vi "Lancing_Presence_Absence.vi"(0 "Ref ROI Parameters":T5={"Ref ROI"={"Global Rectangle"=[], "Contours"=[]}, "Ref ROI Edge Options"={"Edge Polarity"=2, "Kernel Size"=3, "Width"=3, "Minimum Edge Strength"=50.0, "Interpolation Type"=enum."Zero Order", "Data Processing Method"=enum."Average"}, "Ref ROI Line Options"={"Number of Lines"=1, "Type"=enum."Best Edge Rake", "Min. Score"=10.0, "Max. Score"=1000.0, "Orientation"=0.0, "Angle Range"=10.0, "Angle Tolerance"=10.0, "Step Size"=8, "Min. SNR (db)"=0.0, "Min. Points (%)"=25.0, "Hough Iterations"=5}, "Ref ROI Search Direction"=0, "Ref ROI Overlay"=FALSE, "Ref Edge/Point Overlay"=FALSE, "Ref ROI Rake Line Overlay"=FALSE} {"Ref ROI Search Direction" items=["Left to Right", "Right to Left", "Top to Bottom", "Bottom to Top"]; "Ref ROI Line Options"."Min. Points (%)" min=0.0 max=100.0; "Ref ROI Line Options"."Min. SNR (db)" min=0.0; "Ref ROI Line Options"."Max. Score" min=0.0 max=1024.0; "Ref ROI Line Options"."Min. Score" min=0.0 max=1024.0 step=1.0; "Ref ROI Edge Options"."Edge Polarity" items=["All Edges", "Rising Edges", "Falling Edges"]; "Ref ROI Edge Options"."Minimum Edge Strength" format="%.2f"; "Ref ROI Edge Options"."Width" step=2; "Ref ROI Edge Options"."Kernel Size" step=2; "Ref ROI"."Contours"."Type" items=["No Selection", "Point", "Line", "Rectangle", "Oval", "Polygon", "Free", "Annulus", "Unused2", "Unused3", "Broken Line", "Free Hand Line", "Rotated Rectangle"]}, 1 "Calibrated Image":T8, 5 "ROI 1 Parameters":T7={"ROI 1[Before Transformation]"={"Global Rectangle"=[], "Contours"=[]}, "ROI 1 Edge Options"={"Edge Polarity"=2, "Kernel Size"=3, "Width"=3, "Minimum Edge Strength"=50.0, "Interpolation Type"=enum."Zero Order", "Data Processing Method"=enum."Average"}, "ROI 1 Process"=enum."Get First + Last Edge", "ROI 1 Step Size"=4, "ROI 1 Scan Direction"=3, "ROI 1 Overlay"=FALSE, "ROI 1 Rake Line Overlay"=FALSE, "ROI 1 Edge/Point Overlay "=FALSE} {"ROI 1 Scan Direction" items=["Left To Right", "Right To Left", "Top To Bottom", "Bottom To Top"]; "ROI 1 Edge Options"."Edge Polarity" items=["All Edges", "Rising Edges", "Falling Edges"]; "ROI 1 Edge Options"."Minimum Edge Strength" format="%.2f"; "ROI 1 Edge Options"."Width" step=2; "ROI 1 Edge Options"."Kernel Size" step=2}, 7 "ROI 2 Parameters":T6={"ROI 2 Edge Options"={"Edge Polarity"=2, "Kernel Size"=3, "Width"=3, "Minimum Edge Strength"=50.0, "Interpolation Type"=enum."Zero Order", "Data Processing Method"=enum."Average"}, "ROI 2 Scan Direction"=3, "ROI 2 Step Size"=3, "ROI 2 Process"=enum."Get First + Last Edge", "ROI 2 Overlay"=FALSE, "ROI 2 Rake Line Overlay"=FALSE, "ROI 2 Edge/Point Overlay "=FALSE} {"ROI 2 Scan Direction" items=["Left To Right", "Right To Left", "Top To Bottom", "Bottom To Top"]; "ROI 2 Edge Options"."Edge Polarity" items=["All Edges", "Rising Edges", "Falling Edges"]; "ROI 2 Edge Options"."Minimum Edge Strength" format="%.2f"; "ROI 2 Edge Options"."Width" step=2; "ROI 2 Edge Options"."Kernel Size" step=2}, 9 "Image In":T8(plugin-control), 11 "error in (no error)":errorcluster, 12 "Ellipse Center":cluster{"Center X":dbl, "Center Y":dbl}) -> (4 "Points for Arrow Overlay":cluster{"X":sgl, "Y":sgl}[](array[cluster]), 6 "Value":dbl, 8 "Height 2":sgl, 15 "error out":errorcluster)   [LabVIEW 2019, in "Algorithm.lvclass"]
uses:
  FrameworkOverrides/Algorithm.lvclass
  <vilib>/vision/NI_Vision_Development_Module.lvlib
  <vilib>/vision/Measure.llb/Edge Polarity.ctl
  <vilib>/vision/Measure.llb/Edge Options.ctl
  <vilib>/vision/Image Controls.llb/IMAQ Image.ctl
  <vilib>/vision/Measure.llb/Straight Edge Process.ctl
  <vilib>/vision/Measure.llb/Straight Edge Options.ctl
panel:
  out "Height":sgl
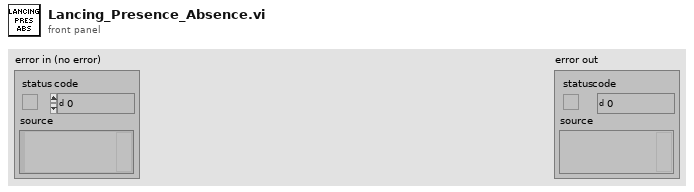
[diagram p1: front panel]
types:
  T1 = typedef "Edge Options.ctl" = cluster{"Edge Polarity":T2, "Kernel Size":u32, "Width":u32, "Minimum Edge Strength":sgl, "Interpolation Type":enum32{"Zero Order", "Bilinear", "Quadratic", "Cubic", "Bilinear Fixed"}, "Data Processing Method":enum32{"Average", "Median"}}
  T2 = typedef "Edge Polarity.ctl" = u32
  T3 = typedef "Straight Edge Options.ctl" = cluster{"Number of Lines":i32, "Type":T4, "Min. Score":dbl, "Max. Score":dbl, "Orientation":dbl, "Angle Range":dbl, "Angle Tolerance":dbl, "Step Size":u32, "Min. SNR (db)":dbl, "Min. Points (%)":dbl, "Hough Iterations":i32}
  T4 = typedef "Straight Edge Process.ctl" = enum32{"First Edge Rake", "Best Edge Rake", "Hough Edge Rake", "First Edge Projection", "Best Edge Projection"}
  T5 = cluster{"Ref ROI":cluster{"Global Rectangle":i32[], "Contours":cluster{"ID":enum32{"External", "Internal"}, "Type":u32, "Coordinates":i32[]}[]}, "Ref ROI Edge Options":T1, "Ref ROI Line Options":T3, "Ref ROI Search Direction":u32, "Ref ROI Overlay":bool, "Ref Edge/Point Overlay":bool, "Ref ROI Rake Line Overlay":bool}
  T6 = cluster{"ROI 2 Edge Options":T1, "ROI 2 Scan Direction":u16, "ROI 2 Step Size":u32, "ROI 2 Process":enum16{"Get First Edge", "Get First + Last Edge", "Get All Edges", "Get Best Edge"}, "ROI 2 Overlay":bool, "ROI 2 Rake Line Overlay":bool, "ROI 2 Edge/Point Overlay ":bool}
  T7 = cluster{"ROI 1[Before Transformation]":cluster{"Global Rectangle":i32[], "Contours":cluster{"Contour Type":u32, "ROI Type":u32, "Points":i32[]}[]}, "ROI 1 Edge Options":T1, "ROI 1 Process":enum16{"Get First Edge", "Get First + Last Edge", "Get All Edges", "Get Best Edge"}, "ROI 1 Step Size":u32, "ROI 1 Scan Direction":u16, "ROI 1 Overlay":bool, "ROI 1 Rake Line Overlay":bool, "ROI 1 Edge/Point Overlay ":bool}
  T8 = typedef "IMAQ Image.ctl" = refnum<image>
  T9 = cluster{"Left":dbl, "Top":dbl, "Right":dbl, "Bottom":dbl, "Angle":dbl}
  T10 = typedef "IMAQ Rectangle" = cluster{"Left":i32, "Top":i32, "Right":i32, "Bottom":i32, "Rotation":dbl}
  T11 = cluster{"Global Rectangle":i32[], "Contours":cluster{"ID":enum32{"External", "Internal"}, "Type":u32, "Coordinates":i32[]}[]}
  T12 = cluster{"ID":enum32{"External", "Internal"}, "Type":u32, "Coordinates":i32[]}[]
  T13 = cluster{"ID":enum32{"External", "Internal"}, "Type":u32, "Coordinates":i32[]}
  T14 = cluster{"Coordinates[0]":i32, "Coordinates[1]":i32, "Coordinates[2]":i32, "Coordinates[3]":i32, "Coordinates[4]":i32}
  T15 = typedef "ROI Descriptor" = cluster{"Global Rectangle":i32[], "Contours":cluster{"ID":enum32{"External", "Internal"}, "Type":u32, "Coordinates":i32[]}[]}
  T16 = cluster{"Global Rectangle":i32[], "Contours":cluster{"Contour Type":u32, "ROI Type":u32, "Points":i32[]}[]}
  T17 = enum16{"Get First Edge", "Get First + Last Edge", "Get All Edges", "Get Best Edge"}
  T18 = cluster{"Contour Type":u32, "ROI Type":u32, "Points":i32[]}[]
  T19 = cluster{"Contour Type":u32, "ROI Type":u32, "Points":i32[]}
  T20 = cluster{"Points[0]":i32, "Points[1]":i32, "Points[2]":i32, "Points[3]":i32, "Points[4]":i32}
  T21 = cluster{"Point1 (Pixels)":cluster{"X":sgl, "Y":sgl}, "Point2 (Pixels)":cluster{"X":sgl, "Y":sgl}, "Point1 (Real-World)":cluster{"X":sgl, "Y":sgl}, "Point2 (Real-World)":cluster{"X":sgl, "Y":sgl}, "Angle (Pixel)":dbl, "Angle (Real-World)":dbl, "Score":dbl, "Straightness":dbl, "Average SNR (db)":dbl, "Calibration Valid":bool}[]
  T22 = typedef "Search Line.ctl" = cluster{"Start Point":cluster{"X":sgl, "Y":sgl}, "End Point":cluster{"X":sgl, "Y":sgl}, "Edge Info":T23[], "Edge Map":dbl[], "Calibration Valid":bool}
  T23 = typedef "Edge New.ctl" = cluster{"Location (Pixel)":cluster{"X":sgl, "Y":sgl}, "Location (Real-World)":cluster{"X":sgl, "Y":sgl}, "Distance (Pixel)":dbl, "Distance (Real-World)":dbl, "Strength":dbl, "Noise":dbl, "Rising?":bool}
  T24 = cluster{"Point1 (Pixels)":cluster{"X":sgl, "Y":sgl}, "Point2 (Pixels)":cluster{"X":sgl, "Y":sgl}, "Point1 (Real-World)":cluster{"X":sgl, "Y":sgl}, "Point2 (Real-World)":cluster{"X":sgl, "Y":sgl}, "Angle (Pixel)":dbl, "Angle (Real-World)":dbl, "Score":dbl, "Straightness":dbl, "Average SNR (db)":dbl, "Calibration Valid":bool}
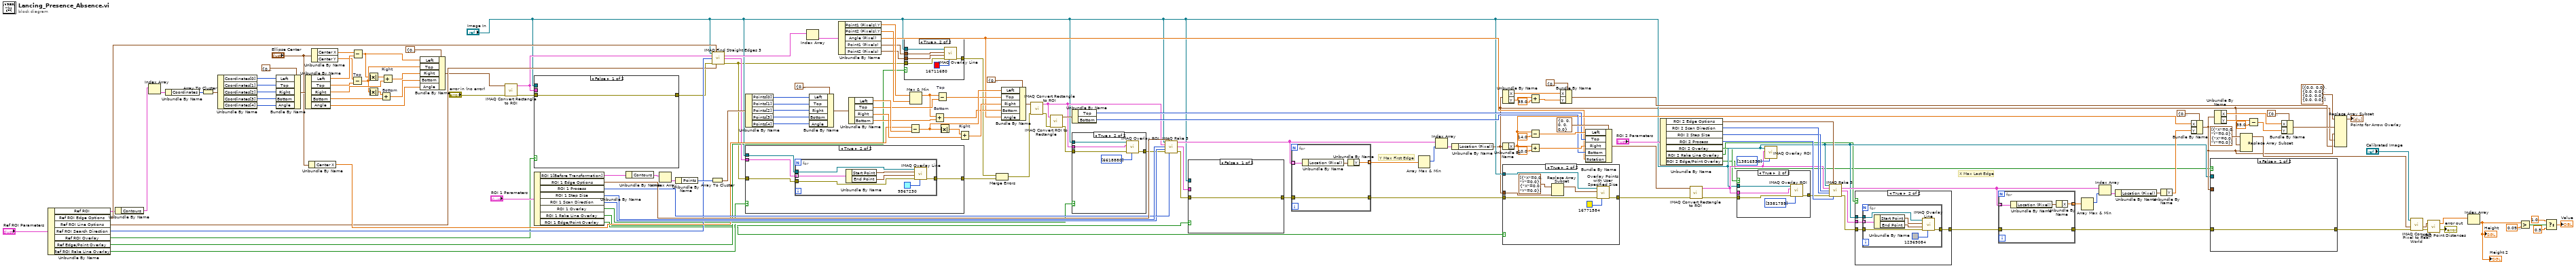
[diagram p0: block diagram]
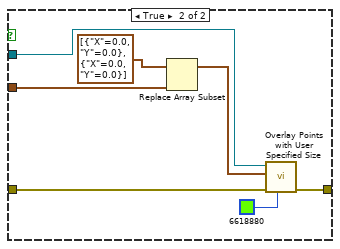
[diagram p2: hidden frame]
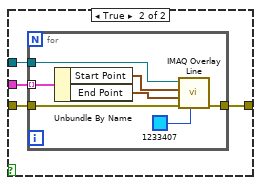
[diagram p5: hidden frame]
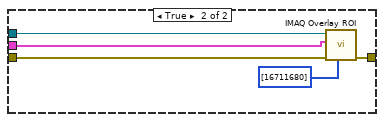
[diagram p10: hidden frame]
diagram:
  # "X Max Last Edge"
  # "Y Max First Edge"
  n1 = Unbundle By Name("Ref ROI Parameters") -> ("Ref ROI"=w45:T11, "Ref ROI Edge Options"=w46:T1, "Ref ROI Line Options"=w47:T3, "Ref ROI Search Direction"=w48:u32, "Ref ROI Overlay"=w30:bool, "Ref Edge/Point Overlay"=w20:bool, "Ref ROI Rake Line Overlay"=w21:bool)
  n2 = Unbundle By Name(w45) -> ("Contours"=w74:T12)
  n3 = Index Array(array=w74) -> (element=w73:T13)  [unwired: 1 in]
  n4 = Unbundle By Name(w73) -> ("Coordinates"=w72:i32[])
  n5 = Array To Cluster(array=w72) -> (cluster=w71:T14)
  n6 = Unbundle By Name(w71) -> ("Coordinates[0]"=w69:i32, "Coordinates[1]"=w68:i32, "Coordinates[2]"=w67:i32, "Coordinates[3]"=w66:i32, "Coordinates[4]"=w65:i32)
  n7 = Bundle By Name(cluster=T9 {"Left"=0.0, "Top"=0.0, "Right"=0.0, "Bottom"=0.0, "Angle"=0.0} ("input cluster"), "Left"=w69, "Top"=w68, "Right"=w67, "Bottom"=w66, "Angle"=w65) -> (w52:T9)
  n8 = Unbundle By Name "Unbundle By Name"(w52) -> ("Left"=w60:dbl, "Top"=w61:dbl, "Right"=w62:dbl, "Bottom"=w63:dbl, "Angle"=w64:dbl)
  n9 = Unbundle By Name("Ellipse Center") -> ("Center X"=w89:dbl)
  n10 = Unbundle By Name("Ellipse Center") -> ("Center X"=w50:dbl, "Center Y"=w51:dbl)
  n11 = Subtract "Top"(x=w51, y=w61) -> (x-y=w57:dbl)
  n12 = Subtract(x=w50, y=w60) -> (x-y=w56:dbl)
  n13 = Absolute Value(x=w56) -> (abs(x)=w53:dbl)
  n14 = Absolute Value(x=w57) -> (abs(x)=w54:dbl)
  n15 = Add "Bottom"(x=w54, y=w63) -> (x+y=w59:dbl)
  n16 = Add "Right"(x=w53, y=w62) -> (x+y=w58:dbl)
  n17 = Bundle By Name(cluster=T9 {"Left"=0.0, "Top"=0.0, "Right"=0.0, "Bottom"=0.0, "Angle"=0.0} ("input cluster"), "Left"=w56, "Top"=w57, "Right"=w58, "Bottom"=w59, "Angle"=w64) -> (w44:T9)
  n18 = call "IMAQ Convert Rectangle to ROI"("error in (no error)"="error in (no error)", "Rectangle"=w44) -> ("error out"=w32:errorcluster, "ROI Descriptor"=w36:T15)  [unwired: 7 in]
  n19 = case shown="False" w30 {
    tunnel: w36 -> [_ w167]
    tunnel: "Image In" -> [_ w165]
    tunnel: w32 -> [w162 w164]
    tunnel: [w162 w163] -> w31
    frame False {
    }
    frame True {
      n20 = call "IMAQ Overlay ROI"("Colors (Green)"=u32[] [16711680], "error in (no error)"=w164, "ROI Descriptor"=w167, "Image"=w165) -> ("error out"=w163:errorcluster)  [unwired: 6 in, 1 out]
    }
  }
  n21 = Unbundle By Name("ROI 1 Parameters") -> ("ROI 1[Before Transformation]"=w41:T16, "ROI 1 Edge Options"=w110:T1, "ROI 1 Process"=w108:T17, "ROI 1 Step Size"=w109:u32, "ROI 1 Scan Direction"=w107:u16, "ROI 1 Overlay"=w26:bool, "ROI 1 Rake Line Overlay"=w13:bool, "ROI 1 Edge/Point Overlay"=w10:bool)
  n22 = Unbundle By Name(w41) -> ("Contours"=w83:T18)
  n23 = Index Array(array=w83) -> (element=w84:T19)  [unwired: 1 in]
  n24 = Unbundle By Name(w84) -> ("Points"=w85:i32[])
  n25 = Array To Cluster(array=w85) -> (cluster=w76:T20)
  n26 = call "IMAQ Find Straight Edges 3"("Image"="Image In", "Edge Options"=w46, "ROI Descriptor"=w36, "Search Direction"=w48, "error in (no error)"=w31, "Line Options"=w47) -> ("Straight Edges"=w40:T21, "Search Lines Information"=w23:T22[], "error out"=w19:errorcluster)  [unwired: 5 in, 2 out]
  n27 = Unbundle By Name "Unbundle By Name"(w76) -> ("Points[0]"=w78:i32, "Points[1]"=w79:i32, "Points[2]"=w80:i32, "Points[3]"=w81:i32, "Points[4]"=w82:i32)
  n28 = case shown="True" w21 {
    tunnel: w23 -> [_ w172]
    tunnel: "Image In" -> [_ w171]
    tunnel: w19 -> [w168 w170]
    tunnel: [w168 w169] -> w17
    frame False {
    }
    frame True {
      n29 = for {
        tunnel: w172 -> [w179] mode=indexing
        tunnel: w171 -> [w176]
        tunnel: w170 -> [w175]
        tunnel: [w174] -> w169
        n30 = Unbundle By Name(w179) -> ("Start Point"=w178:cluster{"X":sgl, "Y":sgl}, "End Point"=w177:cluster{"X":sgl, "Y":sgl})
        n31 = call "IMAQ Overlay Line"("Color"=u32 9567230, "error in (no error)"=w175, "End Point"=w177, "Start Point"=w178, "Image"=w176) -> ("error out"=w174:errorcluster)  [unwired: 5 in, 1 out]
      }
    }
  }
  n32 = Index Array(array=w40) -> (element=w90:T24)  [unwired: 1 in]
  n33 = Bundle By Name(cluster=T9 {"Left"=0.0, "Top"=0.0, "Right"=0.0, "Bottom"=0.0, "Angle"=0.0} ("Measurement ROI-1 Before transformation"), "Left"=w78, "Top"=w79, "Right"=w80, "Bottom"=w81, "Angle"=w82) -> (w75:T9)
  n34 = Unbundle By Name(w90) -> ("Point1 (Pixels).Y"=w88:sgl, "Point2 (Pixels).Y"=w87:sgl, "Angle (Pixel)"=w33:dbl, "Point1 (Pixels)"=w38:cluster{"X":sgl, "Y":sgl}, "Point2 (Pixels)"=w37:cluster{"X":sgl, "Y":sgl})
  n35 = Unbundle By Name(w75) -> ("Left"=w94:dbl, "Top"=w93:dbl, "Right"=w92:dbl, "Bottom"=w91:dbl)
  n36 = case shown="True" w20 {
    tunnel: w38 -> [_ w186]
    tunnel: w37 -> [_ w185]
    tunnel: "Image In" -> [_ w183]
    tunnel: w19 -> [w180 w182]
    tunnel: [w180 w181] -> w18
    frame False {
    }
    frame True {
      n37 = call "IMAQ Overlay Line"("Color"=u32 16711680, "error in (no error)"=w182, "End Point"=w185, "Start Point"=w186, "Image"=w183) -> ("error out"=w181:errorcluster)  [unwired: 5 in, 1 out]
    }
  }
  n38 = Subtract(x=w89, y=w94) -> (x-y=w98:dbl)
  n39 = Max & Min(x=w88, y=w87) -> (max(x,y)=w86:sgl)  [unwired: 1 out]
  n40 = Add "Bottom"(x=w86, y=w91) -> (x+y=w95:dbl)
  n41 = Subtract "Top"(x=w86, y=w93) -> (x-y=w97:dbl)
  n42 = Absolute Value(x=w98) -> (abs(x)=w100:dbl)
  n43 = Add "Right"(x=w100, y=w92) -> (x+y=w96:dbl)
  n44 = Merge Errors(w18, w17) -> (w16:errorcluster)
  n45 = Bundle By Name(cluster=T9 {"Left"=0.0, "Top"=0.0, "Right"=0.0, "Bottom"=0.0, "Angle"=0.0} ("input cluster"), "Left"=w98, "Top"=w97, "Right"=w96, "Bottom"=w95, "Angle"=w33) -> (w42:T9)
  n46 = call "IMAQ Convert Rectangle to ROI"("error in (no error)"=w16, "Rectangle"=w42) -> ("error out"=w29:errorcluster, "ROI Descriptor"=w35:T15)  [unwired: 7 in]
  n47 = call "IMAQ Convert ROI to Rectangle"("error in (no error)"=w29, "ROI Descriptor"=w35) -> ("error out"=w28:errorcluster, "Rectangle"=w156:T10)  [unwired: 7 in]
  n48 = Unbundle By Name(w156) -> ("Top"=w149:i32, "Bottom"=w148:i32)
  n49 = case shown="True" w26 {
    tunnel: w35 -> [_ w191]
    tunnel: "Image In" -> [_ w190]
    tunnel: w28 -> [w187 w189]
    tunnel: [w187 w188] -> w27
    frame False {
    }
    frame True {
      n50 = call "IMAQ Overlay ROI"("Colors (Green)"=u32[] [6618880], "error in (no error)"=w189, "ROI Descriptor"=w191, "Image"=w190) -> ("error out"=w188:errorcluster)  [unwired: 6 in, 1 out]
    }
  }
  n51 = call "IMAQ Rake 3"("Image"="Image In", "Edge Options"=w110, "ROI Descriptor"=w35, "Step Size"=w109, "Scan Direction"=w107, "error in (no error)"=w27, "Process"=w108) -> ("First Edges"=w160:T23[], "Search Lines"=w119:T22[], "error out"=w15:errorcluster)  [unwired: 5 in, 1 out]
  n52 = case shown="False" w13 {
    tunnel: w119 -> [_ w197]
    tunnel: "Image In" -> [_ w196]
    tunnel: w15 -> [w193 w195]
    tunnel: [w193 w194] -> w14
    frame False {
    }
    frame True {
      n53 = for {
        tunnel: w197 -> [w204] mode=indexing
        tunnel: w196 -> [w201]
        tunnel: w195 -> [w199]
        tunnel: [w198] -> w194
        n54 = Unbundle By Name(w204) -> ("Start Point"=w203:cluster{"X":sgl, "Y":sgl}, "End Point"=w202:cluster{"X":sgl, "Y":sgl})
        n55 = call "IMAQ Overlay Line"("Color"=u32 1233407, "error in (no error)"=w199, "End Point"=w202, "Start Point"=w203, "Image"=w201) -> ("error out"=w198:errorcluster)  [unwired: 5 in, 1 out]
      }
    }
  }
  n56 = for {
    tunnel: w160 -> [w208] mode=indexing
    tunnel: [w206] -> w161 mode=indexing
    tunnel: w14 -> [w205]
    tunnel: [w205] -> w12
    n57 = Unbundle By Name(w208) -> ("Location (Pixel)"=w207:cluster{"X":sgl, "Y":sgl})
    n58 = Unbundle By Name(w207) -> ("Y"=w206:sgl)
  }
  n59 = Array Max & Min(array=w161) -> (max index (indices)=w159:i32)  [unwired: 3 out]
  n60 = Index Array(array=w160, index=w159) -> (element=w154:T23)
  n61 = Unbundle By Name(w154) -> ("Location (Pixel)"=w5:cluster{"X":sgl, "Y":sgl})
  n62 = Unbundle By Name(w5) -> ("X"=w133:sgl, "Y"=w132:sgl)
  n63 = Unbundle By Name(w5) -> ("X"=w141:sgl)
  n64 = case shown="True" w10 {
    tunnel: "Image In" -> [_ w215]
    tunnel: w12 -> [w209 w214]
    tunnel: [w209 w213] -> w11
    tunnel: w5 -> [_ w211]
    frame False {
    }
    frame True {
      n65 = Replace Array Subset(array=cluster{"X":sgl, "Y":sgl}[] [{"X"=0.0, "Y"=0.0}, {"X"=0.0, "Y"=0.0}] ("Points"), new element=w211) -> (w212:cluster{"X":sgl, "Y":sgl}[])  [unwired: 1 in]
      n66 = call "Overlay Points with User Specified Size.vi"("Color"=u32 16771584, "error in"=w214, "Points"=w212, "Image In"=w215) -> ("error out"=w213:errorcluster)  [unwired: 6 in, 1 out]
    }
  }
  n67 = Add(x=w132, y=sgl 35.0) -> (x+y=w130:sgl)
  n68 = Subtract(x=w141, y=sgl 14.0) -> (x-y=w151:sgl)
  n69 = Add(x=w141, y=sgl 10.0) -> (x+y=w150:sgl)
  n70 = Bundle By Name(cluster=cluster{"X":sgl, "Y":sgl} {"X"=0.0, "Y"=0.0} ("Location (Pixel)"), "X"=w133, "Y"=w130) -> (w121:cluster{"X":sgl, "Y":sgl})
  n71 = Bundle By Name(cluster=T10 {"Left"=0, "Top"=0, "Right"=0, "Bottom"=0, "Rotation"=0.0} ("Rectangle"), "Left"=w151, "Top"=w149, "Right"=w150, "Bottom"=w148, "Rotation"=w33) -> (w147:T10)
  n72 = Unbundle By Name("ROI 2 Parameters") -> ("ROI 2 Edge Options"=w105:T1, "ROI 2 Scan Direction"=w103:u16, "ROI 2 Step Size"=w102:u32, "ROI 2 Process"=w104:T17, "ROI 2 Overlay"=w9:bool, "ROI 2 Rake Line Overlay"=w8:bool, "ROI 2 Edge/Point Overlay"=w2:bool)
  n73 = call "IMAQ Convert Rectangle to ROI"("error in (no error)"=w11, "Rectangle"=w147) -> ("error out"=w25:errorcluster, "ROI Descriptor"=w34:T15)  [unwired: 7 in]
  n74 = case shown="True" w9 {
    tunnel: "Image In" -> [_ w222]
    tunnel: w34 -> [_ w221]
    tunnel: w25 -> [w217 w219]
    tunnel: [w217 w218] -> w24
    frame False {
    }
    frame True {
      n75 = call "IMAQ Overlay ROI"("Colors (Green)"=u32[] [3381759], "error in (no error)"=w219, "ROI Descriptor"=w221, "Image"=w222) -> ("error out"=w218:errorcluster)  [unwired: 6 in, 1 out]
    }
  }
  n76 = call "IMAQ Overlay ROI"("Colors (Green)"=u32[] [13816530], "ROI Descriptor"=w34, "Image"="Image In") -> ()  [unwired: 7 in, 2 out]
  n77 = call "IMAQ Rake 3"("Image"="Image In", "Edge Options"=w105, "ROI Descriptor"=w34, "Step Size"=w102, "Scan Direction"=w103, "error in (no error)"=w24, "Process"=w104) -> ("Last Edges"=w146:T23[], "Search Lines"=w118:T22[], "error out"=w7:errorcluster)  [unwired: 5 in, 1 out]
  n78 = case shown="True" w8 {
    tunnel: w118 -> [_ w227]
    tunnel: "Image In" -> [_ w226]
    tunnel: w7 -> [w223 w225]
    tunnel: [w223 w224] -> w6
    frame False {
    }
    frame True {
      n79 = for {
        tunnel: w227 -> [w234] mode=indexing
        tunnel: w226 -> [w231]
        tunnel: w225 -> [w229]
        tunnel: [w228] -> w224
        n80 = Unbundle By Name(w234) -> ("Start Point"=w233:cluster{"X":sgl, "Y":sgl}, "End Point"=w232:cluster{"X":sgl, "Y":sgl})
        n81 = call "IMAQ Overlay Line"("Color"=u32 12369084, "error in (no error)"=w229, "End Point"=w232, "Start Point"=w233, "Image"=w231) -> ("error out"=w228:errorcluster)  [unwired: 5 in, 1 out]
      }
    }
  }
  n82 = for {
    tunnel: w146 -> [w238] mode=indexing
    tunnel: [w236] -> w158 mode=indexing
    tunnel: w6 -> [w235]
    tunnel: [w235] -> w4
    n83 = Unbundle By Name(w238) -> ("Location (Pixel)"=w237:cluster{"X":sgl, "Y":sgl})
    n84 = Unbundle By Name(w237) -> ("X"=w236:sgl)
  }
  n85 = Array Max & Min(array=w158) -> (max index (indices)=w157:i32)  [unwired: 3 out]
  n86 = Index Array(array=w146, index=w157) -> (element=w145:T23)
  n87 = Unbundle By Name(w145) -> ("Location (Pixel)"=w144:cluster{"X":sgl, "Y":sgl})
  n88 = Unbundle By Name(w144) -> ("Y"=w142:sgl)
  n89 = Bundle By Name(cluster=cluster{"X":sgl, "Y":sgl} {"X"=0.0, "Y"=0.0} ("Location (Pixel)"), "X"=w141, "Y"=w142) -> (w122:cluster{"X":sgl, "Y":sgl})
  n90 = case shown="False" w2 {
    tunnel: w122 -> [_ w243]
    tunnel: "Image In" -> [_ w242]
    tunnel: w4 -> [w239 w241]
    tunnel: [w239 w240] -> w3
    frame False {
    }
    frame True {
      n91 = Replace Array Subset(array=cluster{"X":sgl, "Y":sgl}[] [{"X"=0.0, "Y"=0.0}, {"X"=0.0, "Y"=0.0}] ("Points"), new element=w243) -> (w246:cluster{"X":sgl, "Y":sgl}[])  [unwired: 1 in]
      n92 = call "Overlay Points with User Specified Size.vi"("Color"=u32 6618880, "error in"=w241, "Points"=w246, "Image In"=w242) -> ("error out"=w240:errorcluster)  [unwired: 6 in, 1 out]
    }
  }
  n93 = Unbundle By Name(w122) -> ("X"=w124:sgl, "Y"=w127:sgl)
  n94 = Replace Array Subset(array=cluster{"X":sgl, "Y":sgl}[] [{"X"=0.0, "Y"=0.0}, {"X"=0.0, "Y"=0.0}] ("Points"), new element #1=w5, new element #2=w122) -> (w139:cluster{"X":sgl, "Y":sgl}[])  [unwired: 2 in]
  n95 = Subtract(x=w127, y=sgl 35.0) -> (x-y=w125:sgl)
  n96 = Bundle By Name(cluster=cluster{"X":sgl, "Y":sgl} {"X"=0.0, "Y"=0.0} ("Location (Pixel)"), "X"=w124, "Y"=w125) -> (w123:cluster{"X":sgl, "Y":sgl})
  n97 = Replace Array Subset(array=cluster{"X":sgl, "Y":sgl}[] [{"X"=0.0, "Y"=0.0}, {"X"=0.0, "Y"=0.0}, {"X"=0.0, "Y"=0.0}, {"X"=0.0, "Y"=0.0}] ("Points"), new element #1=w123, new element #2=w122, new element #3=w5, new element #4=w121) -> (→"Points for Arrow Overlay":cluster{"X":sgl, "Y":sgl}[])  [unwired: 4 in]
  n98 = call "IMAQ Convert Pixel to Real World"("error in (no error)"=w3, "Array of Pixel Coordinates"=w139, "Calibrated Image"="Calibrated Image") -> ("error out"=w138:errorcluster, "Array of Real World Coordinates"=w137:cluster{"X":sgl, "Y":sgl}[])  [unwired: 3 in, 4 out]
  n99 = call "IMAQ Point Distances"("Points"=w137, "error in (no error)"=w138) -> ("Distances"=w136:sgl[], "error out"=→"error out":errorcluster)  [unwired: 3 in]
  n100 = Index Array(array=w136) -> (element=w1:sgl)  [unwired: 1 in]
  "Height" <- w1
  "Height 2" <- w1
  n101 = Greater?(x=w1, y=sgl 0.09) -> (0:w116:bool)
  n102 = Select(t=1.0 ("f"), s=w116, f=0.5 ("t")) -> (s? t:f=→"Value":dbl)
